vi "Decode Data Element Descriptions.vi"(11 "Encoder Data Description":string) -> (3 "Data Encoding":T1)   [LabVIEW 2021, in "CIF_NI_CIPC.lvlib"]
uses:
  CIF_NI_CIPC.lvlib
  TypeDefs/Data Encoding.ctl
  TypeDefs/Alignment.ctl
  <vilib>/CIF Foundation/CIF Utilities/DataTypes/Typedef/Endian.ctl
  TypeDefs/Data Struct Array Info.ctl
  TypeDefs/Data Element.ctl
  <vilib>/Utility/Data Type/Type Definitions/Data Type.ctl
  <vilib>/Utility/Data Type/NI_Data Type.lvlib
  <vilib>/CIF Foundation/CIF Utilities/DataTypes/DataTypes_CIF_U.lvlib
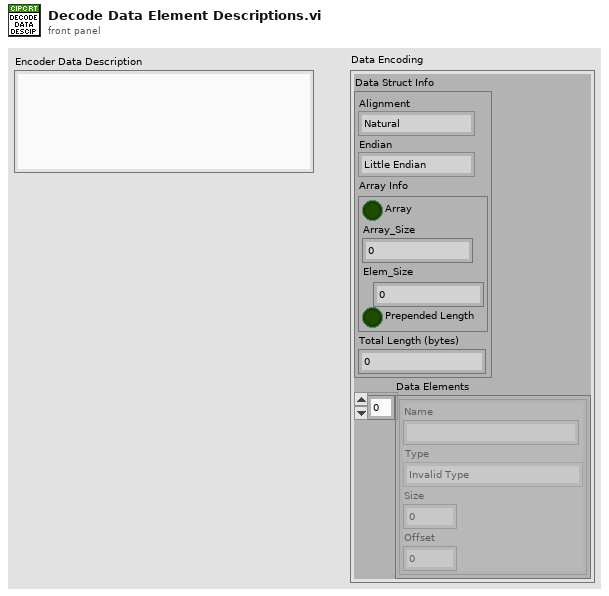
[diagram p1: front panel]
types:
  T1 = typedef "CIF_NI_CIPC.lvlib/Data Encoding.ctl" = cluster{"Data Struct Info":cluster{"Alignment":T2, "Endian":T3, "Array Info":T4, "Total Length (bytes)":i32}, "Data Elements":T5[]}
  T2 = typedef "CIF_NI_CIPC.lvlib/Alignment.ctl" = enum16{"Natural", "Packed"}
  T3 = typedef "DataTypes_CIF_U.lvlib/Endian.ctl" = enum16{"Little Endian", "Big Endian"}
  T4 = typedef "CIF_NI_CIPC.lvlib/Data Struct Array Info.ctl" = cluster{"Array":bool, "Array_Size":i32, "Elem_Size":i32, "Prepended Length":bool}
  T5 = typedef "CIF_NI_CIPC.lvlib/Data Element.ctl" = cluster{"Name":string, "Type":T6, "Size":u32, "Offset":u32}
  T6 = typedef "NI_Data Type.lvlib/Data Type.ctl" = enum8{"Invalid Type", "Void", "I8", "I16", "I32", "I64", "U8", "U16", "U32", "U64", "Single Float", "Double Float", "Extended Float", "Single Complex", "Double Complex", "Extended Complex", "Enum U8", "Enum U16", "Enum U32", "Enum U64", "Single Float With Unit", "Double Float With Unit", "Extended Float With Unit", "Single Complex with Unit", "Double Complex with Unit", "Extended Complex with Unit", "Boolean", "String", "Path", "Picture", "Tag", "Array", "Cluster", "Variant", "LV Variant", "Waveform", "Timestamp", "Digital Waveform", "Digital Data", "ExpressData", "Refnum", "External Data", "VI", "Poly VI", "LabVIEW Class Instance", "Fixed Point", "Set Collection", "Map Collection"}
  T7 = typedef "CIF_NI_CIPC.lvlib/Data Struct Info.ctl" = cluster{"Alignment":T2, "Endian":T3, "Array Info":T4, "Total Length (bytes)":i32}
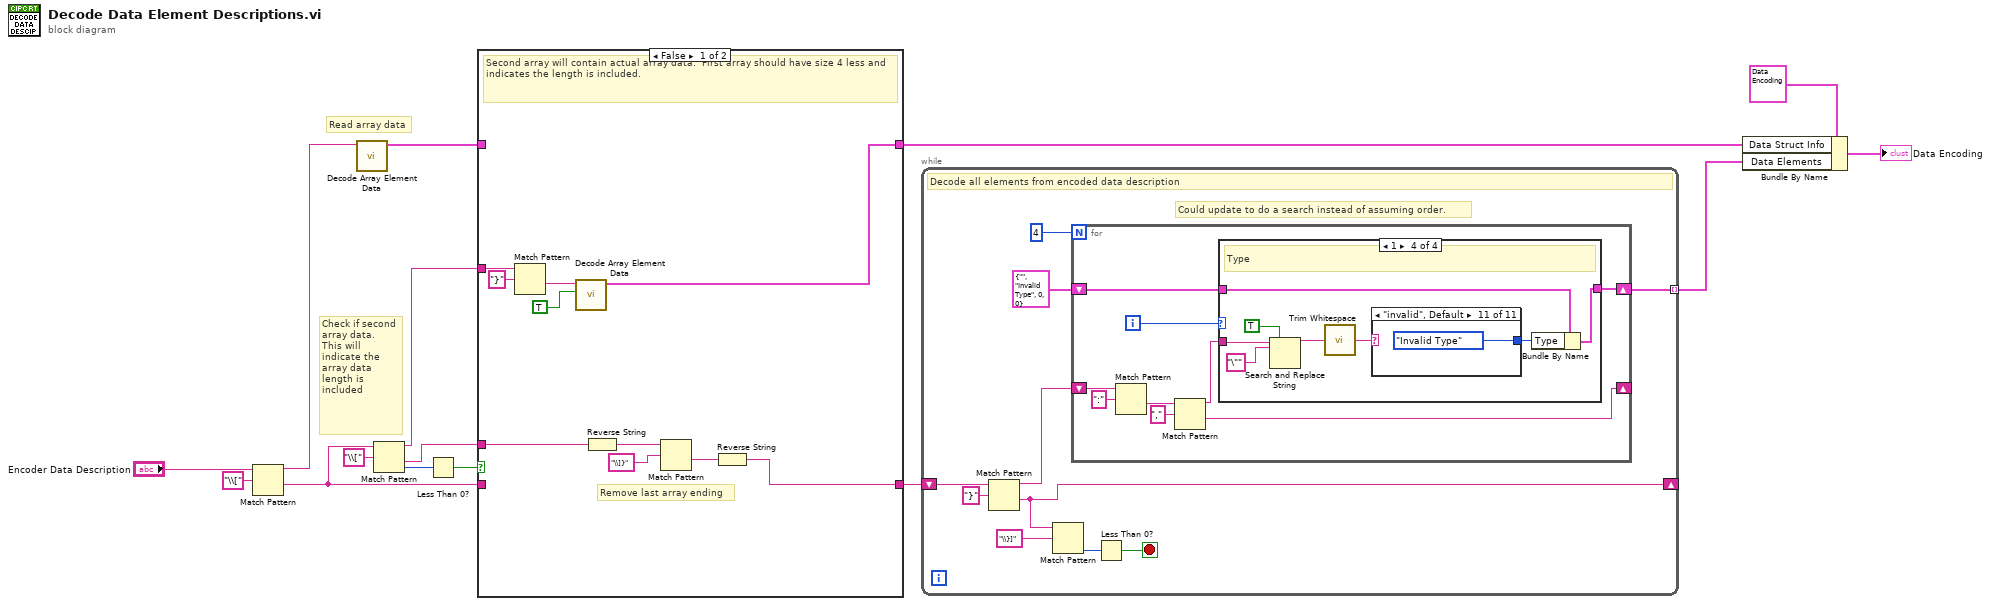
[diagram p0: block diagram]
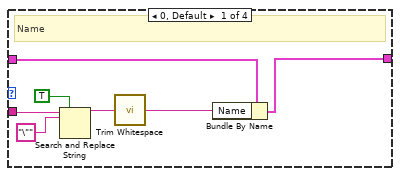
[diagram p3: hidden frame]
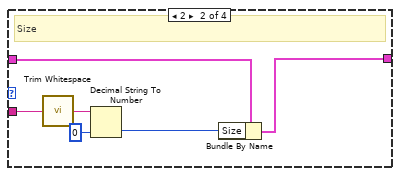
[diagram p4: hidden frame]
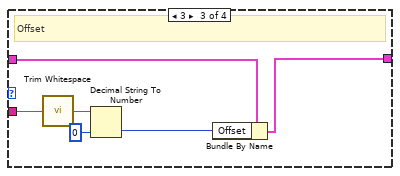
[diagram p5: hidden frame]
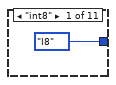
[diagram p6: hidden frame]
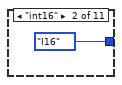
[diagram p7: hidden frame]
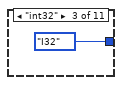
[diagram p8: hidden frame]
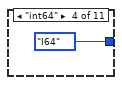
[diagram p9: hidden frame]
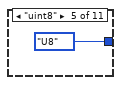
[diagram p10: hidden frame]
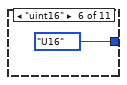
[diagram p11: hidden frame]
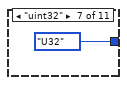
[diagram p12: hidden frame]
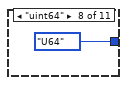
[diagram p13: hidden frame]
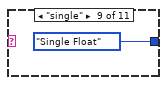
[diagram p14: hidden frame]
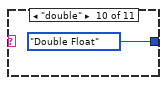
[diagram p15: hidden frame]
diagram:
  # "Check if second array data.  This will indicate the array data length is included"
  # "Read array data"
  n1 = Match Pattern(string="Encoder Data Description", regular expression="\\[") -> (before substring=w13:string, after substring=w9:string)  [unwired: 1 in, 2 out]
  n2 = call "Decode Array Element Data.vi"("Encoder Data Description"=w13) -> ("Array Data Element"=w7:T7)  [unwired: 10 in]
  n3 = Match Pattern(string=w9, regular expression="\\[") -> (before substring=w1:string, after substring=w8:string, offset past match=w11:i32)  [unwired: 1 in, 1 out]
  n4 = Less Than 0?(x=w11) -> (x < 0?=w10:bool)
  n5 = case shown="False" w10 {
    tunnel: w9 -> [_ w27]
    tunnel: w1 -> [w19 _]
    tunnel: [w17 w26] -> w4
    tunnel: w8 -> [w24 _]
    tunnel: w7 -> [_ w26]
    tunnel: [w21 w27] -> w6
    frame False {
      # "Remove last array ending"
      # "Second array will contain actual array data.  First array should have size 4 less and indicates the length is included."
      n6 = Match Pattern(string=w19, regular expression="}") -> (after substring=w18:string)  [unwired: 1 in, 3 out]
      n7 = call "Decode Array Element Data.vi"("Prepended Length"=TRUE, "Encoder Data Description"=w18) -> ("Array Data Element"=w17:T7)  [unwired: 9 in]
      n8 = Reverse String(1:w24) -> (0:w23:string)
      n9 = Match Pattern(string=w23, regular expression="\\]}") -> (after substring=w22:string)  [unwired: 1 in, 3 out]
      n10 = Reverse String(1:w22) -> (0:w21:string)
    }
    frame True {
      # "No second array, no array data length"
    }
  }
  n11 = while {
    shift-right: [w33] -> _
    shift-left: w6 -> [w37]
    tunnel: [w28] -> w3 mode=indexing
    stop <- w35 stop-if-true
    # "Could update to do a search instead of assuming order."
    # "Decode all elements from encoded data description"
    n12 = Match Pattern(string=w37, regular expression="}") -> (before substring=w31:string, after substring=w33:string)  [unwired: 1 in, 2 out]
    n13 = Match Pattern(string=w33, regular expression="\\}]") -> (offset past match=w32:i32)  [unwired: 1 in, 3 out]
    n14 = for {
      N: 4 -> [_]
      shift-right: [w42] -> _
      shift-left: w31 -> [w43]
      shift-right: [w38] -> w28
      shift-left: T5 {"Name"="", "Type"=enum."Invalid Type", "Size"=0, "Offset"=0} -> [w40]
      i -> [w39]
      n15 = Match Pattern(string=w43, regular expression=":") -> (after substring=w45:string)  [unwired: 1 in, 3 out]
      n16 = Match Pattern(string=w45, regular expression=",") -> (before substring=w41:string, after substring=w42:string)  [unwired: 1 in, 2 out]
      n17 = case shown="1" w39 {
        tunnel: w41 -> [w53 w57 w63 w73]
        tunnel: w40 -> [w49 w59 w65 w69]
        tunnel: [w48 w58 w64 w68] -> w38
        frame 0, Default {
          # "Name"
          n18 = Search and Replace String(replace all?=TRUE ("replace all? (F)"), input string=w53, search string="\"") -> (result string=w51:string)  [unwired: 5 in, 3 out]
          n19 = call <vilib>:"Trim Whitespace.vi"("string"=w51) -> ("trimmed string"=w47:string)  [unwired: 1 in]
          n20 = Bundle By Name(cluster=w49, "Name"=w47) -> (w48:T5)
        }
        frame 2 {
          # "Size"
          n21 = call <vilib>:"Trim Whitespace.vi"("string"=w57) -> ("trimmed string"=w56:string)  [unwired: 1 in]
          n22 = Decimal String To Number(string=w56, default (0L)=u32 0 ("default (0 I32)")) -> (number=w54:u32)  [unwired: 1 in, 1 out]
          n23 = Bundle By Name(cluster=w59, "Size"=w54) -> (w58:T5)
        }
        frame 3 {
          # "Offset"
          n24 = call <vilib>:"Trim Whitespace.vi"("string"=w63) -> ("trimmed string"=w62:string)  [unwired: 1 in]
          n25 = Decimal String To Number(string=w62, default (0L)=u32 0 ("default (0 I32)")) -> (number=w60:u32)  [unwired: 1 in, 1 out]
          n26 = Bundle By Name(cluster=w65, "Offset"=w60) -> (w64:T5)
        }
        frame 1 {
          # "Type"
          n27 = Search and Replace String(replace all?=TRUE ("replace all? (F)"), input string=w73, search string="\"") -> (result string=w71:string)  [unwired: 5 in, 3 out]
          n28 = call <vilib>:"Trim Whitespace.vi"("string"=w71) -> ("trimmed string"=w67:string)  [unwired: 1 in]
          n29 = case shown="\"invalid\", Default" w67 {
            tunnel: [Data_Type."I8" ("Type") Data_Type."I16" ("Type") Data_Type."I32" ("Type") Data_Type."I64" ("Type") Data_Type."U8" ("Type") Data_Type."U16" ("Type") Data_Type."U32" ("Type") Data_Type."U64" ("Type") Data_Type."Single Float" ("Type") Data_Type."Double Float" ("Type") Data_Type."Invalid Type" ("Type")] -> w66
            frame "int8" {
            }
            frame "int16" {
            }
            frame "int32" {
            }
            frame "int64" {
            }
            frame "uint8" {
            }
            frame "uint16" {
            }
            frame "uint32" {
            }
            frame "uint64" {
            }
            frame "single" {
            }
            frame "double" {
            }
            frame "invalid", Default {
            }
          }
          n30 = Bundle By Name(cluster=w69, "Type"=w66) -> (w68:T5)
        }
      }
    }
    n31 = Less Than 0?(x=w32) -> (x < 0?=w35:bool)
  }
  n32 = Bundle By Name(cluster=T1 {"Data Struct Info"={"Alignment"=enum."Natural", "Endian"=enum."Little Endian", "Array Info"={"Array"=FALSE, "Array_Size"=0, "Elem_Size"=0, "Prepended Length"=FALSE}, "Total Length (bytes)"=0}, "Data Elements"=[]} ("Data Encoding 2"), "Data Struct Info"=w4, "Data Elements"=w3) -> (→"Data Encoding":T1)
